vi "H5Tget_member_class.vi"(6 "error in (no error)":errorcluster, 8 "Member Number":u32, 9 "HDF5 Type Ref":T1) -> (0 "error out":errorcluster, 2 "class":i32(ring) items=["H5T_NO_CLASS"=-1, "H5T_INTEGER"=0, "H5T_FLOAT"=1, "H5T_TIME"=2, "H5T_STRING"=3, "H5T_BITFIELD"=4, "H5T_OPAQUE"=5, "H5T_COMPOUND"=6, "H5T_REFERENCE"=7, "H5T_ENUM"=8, "H5T_VLEN"=9, "H5T_ARRAY"=10], 3 "HDF5 Type Ref out":T1)   [LabVIEW 2017]
doc: "Returns datatype class of compound datatype member."
uses:
  <vilib>/UPVI/lvhdf5/library.llb/HDF5 Ref.ctl
  <vilib>/UPVI/lvhdf5/hdf5.dll
panel:
  # "LVHDF5 Toolkit\nCopyright (c) 2005-2013 by Jason D. Sommerville\nCopyright (c) 2014 by UPVI, LLC.\n\nThis use and distribution of this file is governed by the terms found in \nLICENSE.txt distributed with this toolkit and installed at\n <user.lib>\\_lvhdf5\\LICENSE.txt"
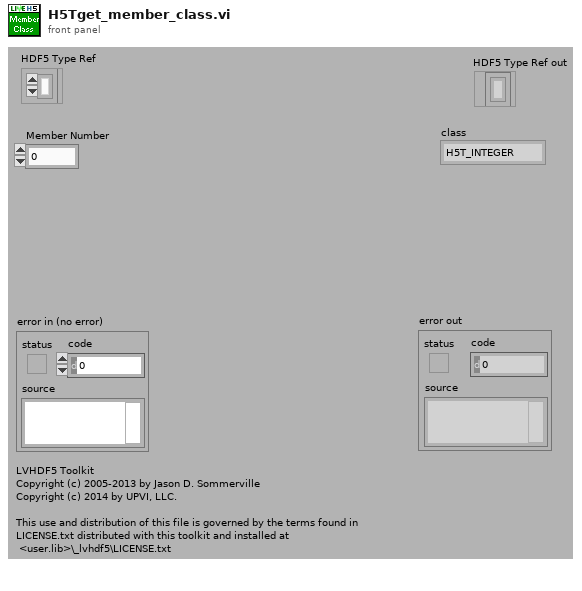
[diagram p1: front panel]
types:
  T1 = typedef "HDF5 Ref.ctl" = refnum<k1>
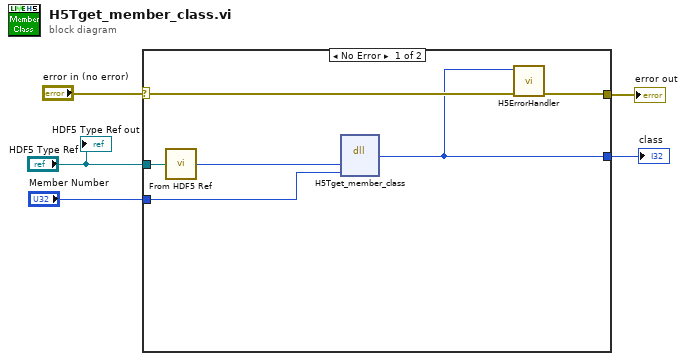
[diagram p0: block diagram]
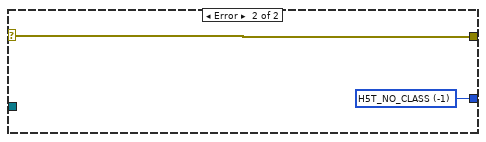
[diagram p2: hidden frame]
diagram:
  n1 = case shown="No Error" "error in (no error)" {
    selector: "error in (no error)" -> [w11 w13]
    tunnel: [w10 w13] -> w4
    tunnel: "HDF5 Type Ref" -> [w9 _]
    tunnel: [w7 w12] -> w2
    tunnel: "Member Number" -> [w6 _]
    frame No Error {
      n2 = call <vilib>:"From HDF5 Ref.vi"("HDF5 Ref"=w9) -> ("I32"=w8:i32)
      n3 = dll-call lib="C:/Program Files/National Instruments/LabVIEW 2017/vi.lib/UPVI/lvhdf5/hdf5.dll" fn="H5Tget_member_class"("type_id"=w8, "member_no"=w6) -> (w7:i32)  [unwired: 5 in, 2 out]
      n4 = call <vilib>:"H5ErrorHandler.vi"("error in (no error)"=w11, "herr_t"=w7) -> ("error out"=w10:errorcluster)  [unwired: 3 in, 4 out]
    }
    frame Error {
      w12 = -1 items=["H5T_NO_CLASS"=-1, "H5T_INTEGER"=0, "H5T_FLOAT"=1, "H5T_TIME"=2, "H5T_STRING"=3, "H5T_BITFIELD"=4, "H5T_OPAQUE"=5, "H5T_COMPOUND"=6, "H5T_REFERENCE"=7, "H5T_ENUM"=8, "H5T_VLEN"=9, "H5T_ARRAY"=10] ("class")
    }
  }
  "error out" <- w4
  "class" <- w2
  "HDF5 Type Ref out" <- "HDF5 Type Ref"
